vi "Shutdown.vi"(8 "error in (no error)":errorcluster, 11 "View in":refnum<class "View.lvclass">) -> (0 "error out":errorcluster, 3 "View out":refnum<class "View.lvclass">)   [LabVIEW 2020, in "Page2.lvlib" / "View.lvclass"]
uses:
  View.lvclass
  View.lvclass/View.ctl
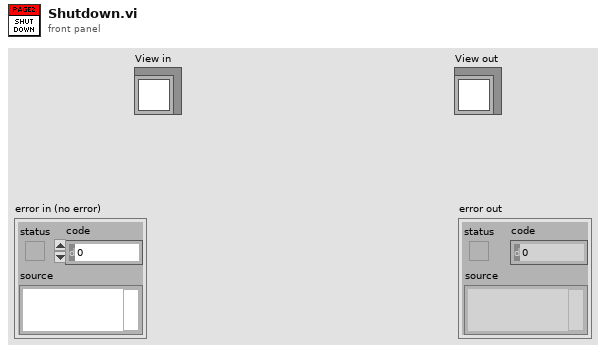
[diagram p1: front panel]
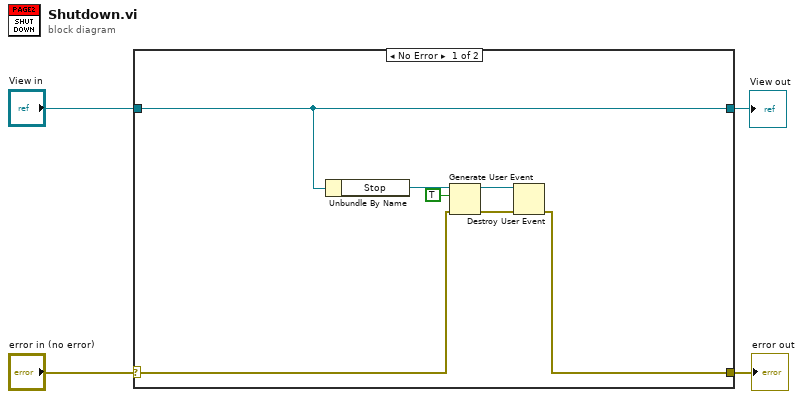
[diagram p0: block diagram]
diagram:
  n1 = case shown="No Error" "error in (no error)" {
    selector: "error in (no error)" -> [w7 w13]
    tunnel: [w5 w13] -> w3
    tunnel: [w11 w12] -> w2
    tunnel: "View in" -> [w11 w12]
    frame No Error {
      n2 = Unbundle By Name(w11) -> ("Stop"=w10:refnum<user-event>)
      n3 = Generate User Event(user event=w10, event data cluster=TRUE ("event data"), error in=w7) -> (user event out=w9:refnum<user-event>, error out=w6:errorcluster)  [unwired: 1 in]
      n4 = Destroy User Event(user event=w9, error in=w6) -> (error out=w5:errorcluster)
    }
    frame Error {
    }
  }
  "error out" <- w3
  "View out" <- w2
